vi "Image Data to RGB Channel.vi"(8 "错误输入":errorcluster, 10 "模式":enum16{"Red", "Green", "Blue"}(ring), 11 "image data In":T1 caption="输入图像数据") -> (0 "错误输出":errorcluster, 3 "image data Out":T1 caption="输出图像数据")   [LabVIEW 2011]
uses:
  <vilib>/picture/picture.llb/imagedata.ctl
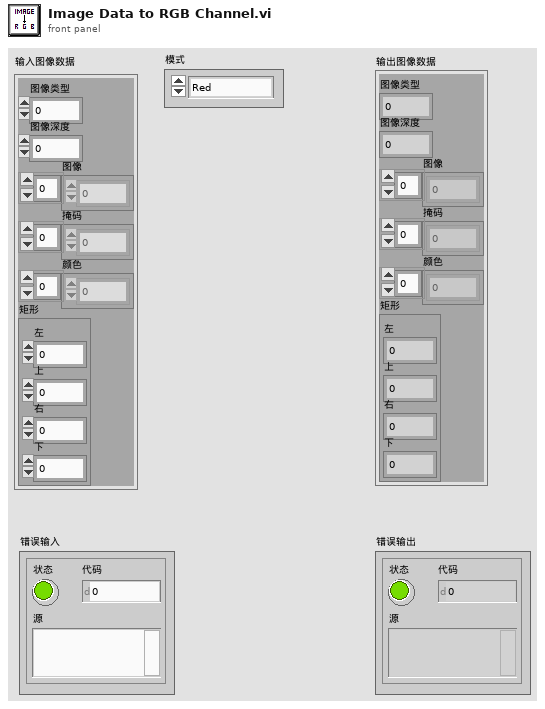
[diagram p1: front panel]
types:
  T1 = typedef "imagedata.ctl" = cluster{"image type":i32, "image depth":i32, "image":u8[], "mask":u8[], "colors":u32[], "Rectangle":cluster{"left":i16, "top":i16, "right":i16, "bottom":i16}}
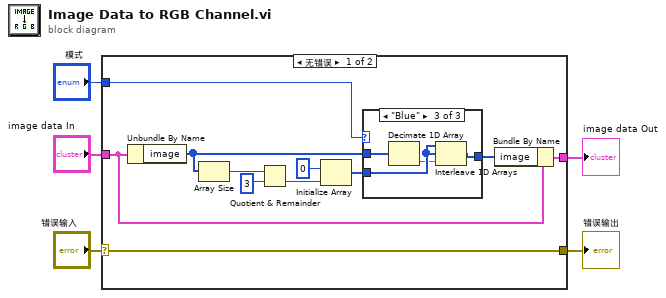
[diagram p0: block diagram]
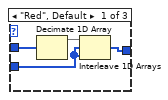
[diagram p2: hidden frame]
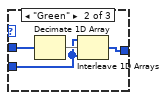
[diagram p3: hidden frame]
diagram:
  n1 = case shown="无错误" "错误输入" {
    selector: "错误输入" -> [w8 w29]
    tunnel: "image data In" -> [w10 _]
    tunnel: [w9 _] -> w4
    tunnel: [w8 w29] -> w2
    tunnel: "模式" -> [w6 _]
    frame No Error {
      n2 = Unbundle By Name(w10) -> ("image"=w7:u8[])
      n3 = Array Size(array=w7) -> (size(s)=w16:i32)
      n4 = Quotient & Remainder(x=w16, y=3) -> (floor(x/y)=w14:i32)  [unwired: 1 out]
      n5 = Initialize Array(u8 0, w14) -> (w11:u8[])
      n6 = case shown="\"Blue\"" w6 {
        tunnel: [w20 w24 w28] -> w12
        tunnel: w11 -> [w17 w21 w26]
        tunnel: w7 -> [w19 w23 w27]
        frame "Red", Default {
          n7 = Decimate 1D Array(w19) -> (w18:u8[])  [unwired: 2 out]
          n8 = Interleave 1D Arrays(w18, w17, w17) -> (w20:u8[])
        }
        frame "Green" {
          n9 = Decimate 1D Array(w23) -> (w22:u8[])  [unwired: 2 out]
          n10 = Interleave 1D Arrays(w21, w22, w21) -> (w24:u8[])
        }
        frame "Blue" {
          n11 = Decimate 1D Array(w27) -> (w25:u8[])  [unwired: 2 out]
          n12 = Interleave 1D Arrays(w26, w26, w25) -> (w28:u8[])
        }
      }
      n13 = Bundle By Name(cluster=w10, "image"=w12) -> (w9:T1)
    }
    frame Error {
    }
  }
  "image data Out" <- w4
  "错误输出" <- w2
